vi "AlGaAs_string_v00.vi"(1 "Ga run":bool, 2 "RGa":dbl, 3 "Al run":bool, 4 "RAl":dbl) -> (0 "result":string)   [LabVIEW 2011]
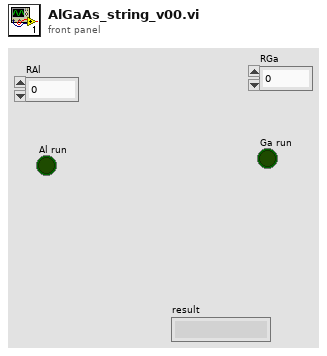
[diagram p1: front panel]
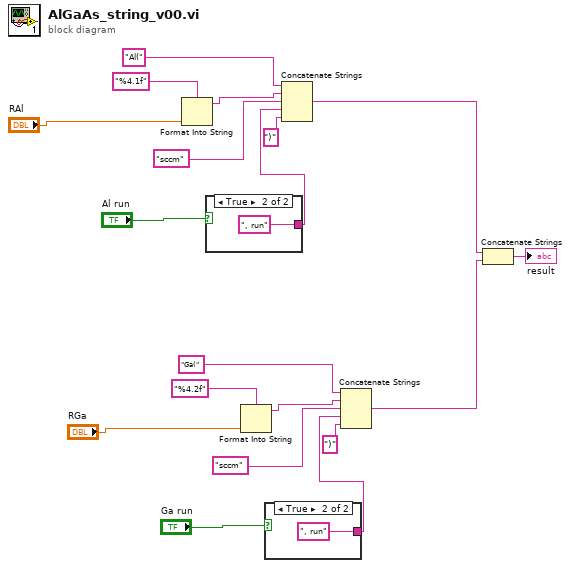
[diagram p0: block diagram]
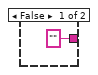
[diagram p2: hidden frame]
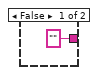
[diagram p3: hidden frame]
diagram:
  n1 = Format Into String(format string="%4.1f", "RAl") -> (resulting string=w15:string)  [unwired: 2 in, 1 out]
  n2 = case shown="True" "Al run" {
    tunnel: ["" ", run"] -> w17
    frame False {
    }
    frame True {
    }
  }
  n3 = Format Into String(format string="%4.2f", "RGa") -> (resulting string=w7:string)  [unwired: 2 in, 1 out]
  n4 = case shown="True" "Ga run" {
    tunnel: ["" ", run"] -> w9
    frame False {
    }
    frame True {
    }
  }
  n5 = Concatenate Strings("Al(" ("string"), w15, "sccm" ("string"), w17, ")" ("string")) -> (w3:string)
  n6 = Concatenate Strings("Ga(" ("string"), w7, "sccm" ("string"), w9, ")" ("string")) -> (w2:string)
  n7 = Concatenate Strings(w3, w2) -> (→"result":string)
